vi "Build Register Status Message.vi"(0 "Target CSM":string, 5 "Source CSM (* as Default)":string="*", 7 "Status":string, 9 "API (If \"\", Same As \"Status\")":string) -> (6 "CSM Message String":string)   [LabVIEW 2017, in "Communicable State Machine.lvlib"]
doc: "#### Build Register Status Message.vi\n\nConcatenates a register status operation message string, with the following format:\n\n //[source-state]@[source-module] >> [response-message]@[response-module] -><register>\n status @ Source >> API @ Target -><register>\n\nExample: Add the download completion message of the downloader module, binding it to the start play API of the player module.\n\n // Bind the download completion message of the downloader module to the start play API of the player module.\n DownloadFinished@Downloader >> StartPlay@Player -><register>\n // When executing the message in the player module, Player can be omitted.\n DownloadFinished@Downloader >> StartPlay -><register>\n // When multiple modules have download completion messages, use * to indicate that all modules' messages are bound to the start play API of the player module.\n DownloadFinished@* >> StartPlay@Player -><register>\n\n> [!NOTE] Message Concatenation API\n> This type of API does not directly send messages, it only concatenates message strings. The strings need to be incorporated into the CSM's state queue and then sent and executed in Parse State Queue++.vi.\n> If you are familiar with CSM rules, you can skip using this type of API and directly type the corresponding message strings and operation strings in the text.\n\n\n<b>Controls</b>\n- <b>Target CSM</b>: The name of the CSM module subscribing to the status.\n- <b>Source CSM (* as Default)</b>: The name of the CSM module issuing the status.\n- <b>Status</b>: The registered status.\n- <b>API (if \"\", same as Status)</b>: The API name that the subscribing status module responds to.\n\n<b>Indicators</b>\n- <b>CSM Message String</b>: The concatenated CSM message string."
uses:
  Communicable State Machine.lvlib
  _Shared/CSM Shared.lvlib
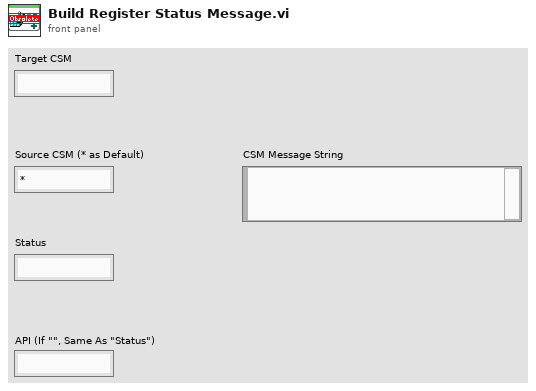
[diagram p1: front panel]
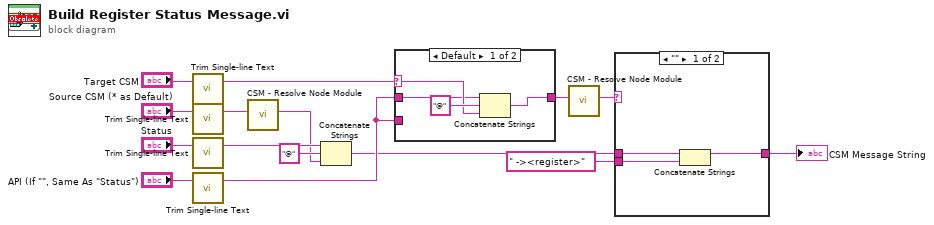
[diagram p0: block diagram]
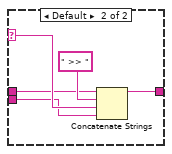
[diagram p2: hidden frame]
diagram:
  n1 = call "Trim Single-line Text.vi"("single-line text"="Target CSM") -> ("trimed text"=w6:string)  [unwired: 2 in]
  n2 = call "Trim Single-line Text.vi"("single-line text"="Source CSM (* as Default)") -> ("trimed text"=w8:string)  [unwired: 2 in]
  n3 = call "Trim Single-line Text.vi"("single-line text"="Status") -> ("trimed text"=w10:string)  [unwired: 2 in]
  n4 = call "Trim Single-line Text.vi"("single-line text"="API (If \"\", Same As \"Status\")") -> ("trimed text"=w7:string)  [unwired: 2 in]
  n5 = call "CSM - Resolve Node Module.vi"("Node Name"=w8) -> ("CSM Module Name"=w2:string)  [unwired: 10 in]
  n6 = Concatenate Strings(w10, "@" ("string"), w2) -> (w4:string)
  n7 = case shown="Default" w6 {
    selector: w6 -> [w17 _]
    tunnel: [w18 w20] -> w5
    tunnel: w7 -> [w16 w20]
    tunnel: w7 -> [_ _]
    frame Default {
      n8 = Concatenate Strings(w16, "@" ("string"), w17) -> (w18:string)
    }
    frame "" {
    }
  }
  n9 = call "CSM - Resolve Node Module.vi"("Node Name"=w5) -> ("CSM Module Name"=w1:string)  [unwired: 10 in]
  n10 = case shown="\"\"" w1 {
    selector: w1 -> [_ w26]
    tunnel: [w21 w28] -> w15
    tunnel: w4 -> [w23 w25]
    tunnel: " -><register>" ("string") -> [w22 w24]
    frame "" {
      n11 = Concatenate Strings(w23, w22) -> (w21:string)
    }
    frame Default {
      n12 = Concatenate Strings(w25, " >> " ("string"), w26, w24) -> (w28:string)
    }
  }
  "CSM Message String" <- w15
